vi "DriveForTime.vi"() -> ()   [LabVIEW 2018]
uses:
  Framework/Robot Global Data.vi
panel:
  in  "NoWait":bool
  in  "Seconds":dbl
  in  "RightSpeed":dbl
  in  "LeftSpeed":dbl
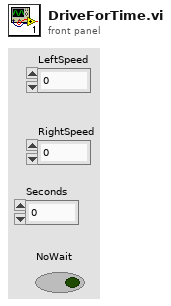
[diagram p1: front panel]
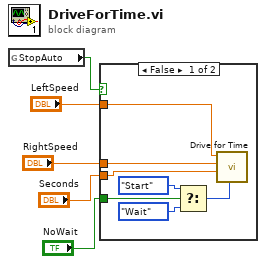
[diagram p0: block diagram]
diagram:
  n1 = global read "Robot Global Data.vi" "StopAuto"() -> (w5:bool)
  n2 = case shown="False" w5 {
    tunnel: "LeftSpeed" -> [w12 _]
    tunnel: "RightSpeed" -> [w11 _]
    tunnel: "Seconds" -> [w10 _]
    tunnel: "NoWait" -> [w9 _]
    frame False {
      n3 = Select(t=enum16{"Start", "Wait"}."Start" ("Synchronization"), s=w9, f=enum16{"Start", "Wait"}."Wait" ("Synchronization")) -> (s? t:f=w8:enum16{"Start", "Wait"})
      n4 = call "Drive for Time.vi"("Synchronization"=w8, "Seconds"=w10, "Right Speed"=w11, "Left Speed"=w12) -> ()  [unwired: 7 in, 1 out]
    }
    frame True {
    }
  }
